vi "Mobility-Vt-Used Pts_Saturation_AMZ_StdDEV_Edit.vi"(0 "Vg Used":dbl[](array[numeric]), 1 "Length":dbl, 3 "Width":dbl, 5 "Sat Id Used":dbl[](array[numeric]), 9 "Dielectric (d)":dbl, 12 "Dielectric Const":dbl) -> (4 "Mobility":dbl, 6 "Vt":dbl, 10 "Capacitance":dbl, 15 "Threshold Voltage Error":dbl)   [LabVIEW 2015]
uses:
  <vilib>/Analysis/6fits.llb/Confidence Interval (Linear).vi
  <vilib>/Analysis/NI_AALPro.lvlib
panel:
  out "delta slope":dbl
  out "delta intercept":dbl
  out "residue":dbl
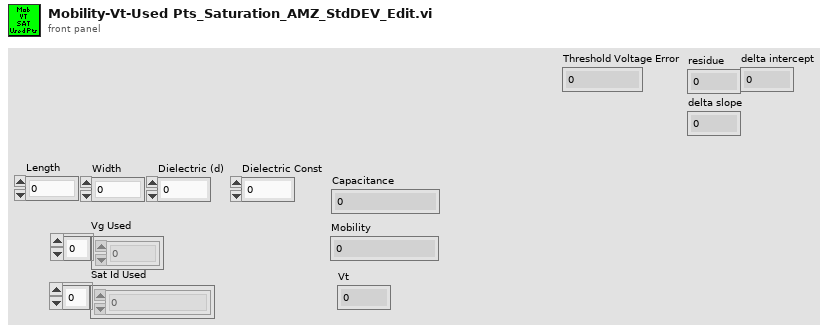
[diagram p1: front panel]
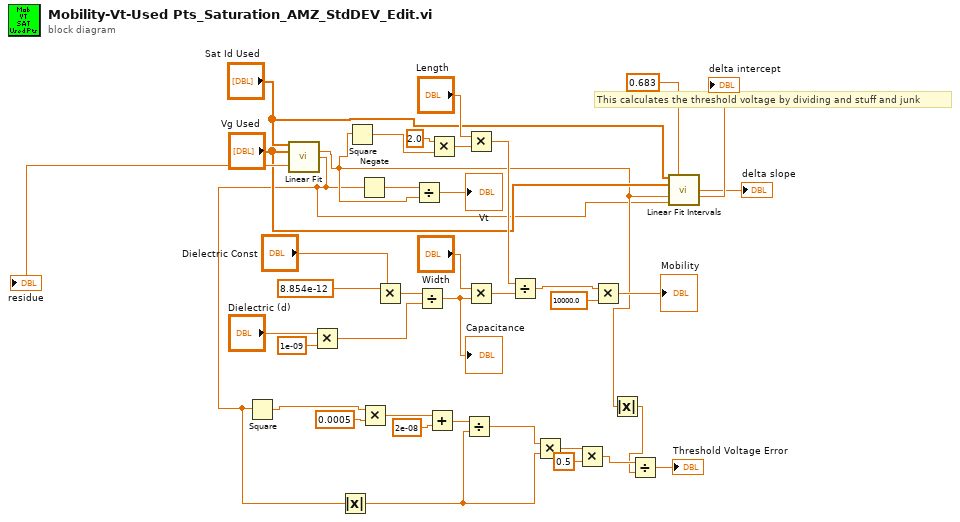
[diagram p0: block diagram]
diagram:
  # "This calculates the threshold voltage by dividing and stuff and junk"
  n1 = call <vilib>:"Linear Fit.vi"("Y"="Sat Id Used", "X"="Vg Used") -> ("slope"=w2:dbl, "intercept"=w1:dbl, "residue"=→"residue":dbl)  [unwired: 9 in, 2 out]
  n2 = Square(x=w1) -> (x^2=w12:dbl)
  n3 = Multiply(x="Dielectric (d)", y=1e-09) -> (x*y=w38:dbl)
  n4 = Absolute Value(x=w1) -> (abs(x)=w8:dbl)
  n5 = Square(x=w2) -> (x^2=w9:dbl)
  n6 = Negate(x=w1) -> (-x=w24:dbl)
  n7 = Multiply(x=w12, y=0.0005) -> (x*y=w20:dbl)
  n8 = Multiply(x=8.854e-12, y="Dielectric Const") -> (x*y=w39:dbl)
  n9 = Divide(x=w24, y=w2) -> (x/y=→"Vt":dbl)
  n10 = Divide(x=w39, y=w38) -> (x/y=w23:dbl)
  "Capacitance" <- w23
  n11 = Add(x=w20, y=2e-08) -> (x+y=w18:dbl)
  n12 = Multiply(x=2.0, y=w9) -> (x*y=w32:dbl)
  n13 = Divide(x=w18, y=w8) -> (x/y=w17:dbl)
  n14 = Multiply(x="Length", y=w32) -> (x*y=w31:dbl)
  n15 = Multiply(x="Width", y=w23) -> (x*y=w30:dbl)
  n16 = Divide(x=w31, y=w30) -> (x/y=w28:dbl)
  n17 = Multiply(x=w17, y=w8) -> (x*y=w16:dbl)
  n18 = Multiply(x=w16, y=0.5) -> (x*y=w14:dbl)
  n19 = Multiply(x=w28, y=10000.0) -> (x*y=→"Mobility":dbl)
  n20 = Absolute Value(x=w2) -> (abs(x)=w11:dbl)
  n21 = Divide(x=w14, y=w11) -> (x/y=→"Threshold Voltage Error":dbl)
  n22 = call-poly <vilib>:"Linear Fit Intervals.vi"("Y"="Sat Id Used", "confidence level"=0.683, "X"="Vg Used", "slope"=w2, "intercept"=w1) -> ("delta slope"=→"delta slope":dbl, "delta intercept"=→"delta intercept":dbl)  [unwired: 6 in, 3 out]
